vi "Tosca-Clear Digital Outputs.vi"(0 "Config path":path, 11 "error in (no error)":errorcluster) -> (15 "error out":errorcluster)   [LabVIEW 2020]
uses:
  TTL VIs/Device Classes/Base Class/TTLControlledDevice.lvclass
  TTL VIs/Device Classes/Base Class/TTLControlledDevice.lvclass/TTLControlledDevice.ctl
  TTL VIs/Device Classes/Base Class/Read Line.vi
  <vilib>/DAQmx/write.llb/DAQmx Write (Digital 1D Bool 1Chan 1Samp).vi
  epl-vi-lib/Utility VIs/File IO VIs/Configuration File Wrapper VIs/Config-Read Key (string).vi
  <vilib>/DAQmx/create/channels.llb/DAQmx Create Channel (DO-Digital Output).vi
  <vilib>/DAQmx/miscellaneous.llb/DAQmx Fill In Error Info.vi
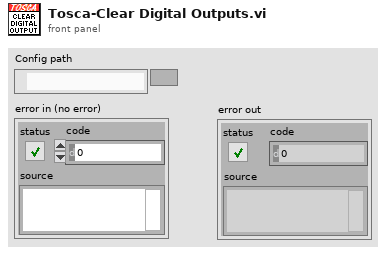
[diagram p1: front panel]
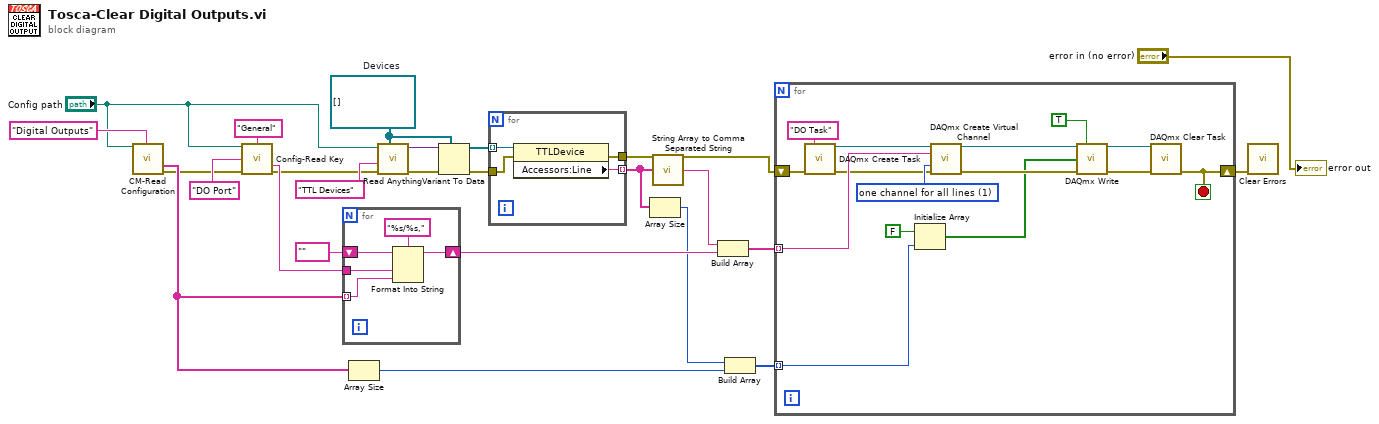
[diagram p0: block diagram]
diagram:
  w15 = refnum<class "TTLControlledDevice.lvclass">[] []  # Devices
  n1 = call "CM-Read Configuration.vi"("Connection File Path"="Config path", "Section"="Digital Outputs") -> ("Devices"=w2:string[], "error out"=w1:errorcluster)  [unwired: 9 in, 3 out]
  n2 = call-poly "Config-Read Key.vi"("configuration file path"="Config path", "section"="General", "key"="DO Port", "error in (no error)"=w1) -> ("value"=w21:string, "error out"=w18:errorcluster)  [unwired: 8 in, 2 out]
  n3 = for {
    tunnel: w2 -> [w26] mode=indexing
    shift-right: [w28] -> w22
    shift-left: tag "" ("DAQmx Physical Channel") -> [w29]
    tunnel: w21 -> [w27]
    n4 = Format Into String(format string="%s/%s,", initial string=w29, w27, w26) -> (resulting string=w28:string)  [unwired: 1 in, 1 out]
  }
  n5 = Array Size(array=w2) -> (size(s)=w20:i32)
  n6 = call "Read Anything.vi"("Type of Anything"=w15, "Error In"=w18, "Section Name (Name of \"Type of Anything\")"="TTL Devices" ("Section Name (Name of \"Type of Anything\")"), "Path (dialog)"="Config path") -> ("Error Out"=w17:errorcluster, "Anything"=w16:variant)  [unwired: 5 in, 1 out]
  n7 = Variant To Data(error in=w17, type=w15, Variant=w16) -> (data=w13:refnum<class "TTLControlledDevice.lvclass">[], error out=w14:errorcluster)
  n8 = for {
    tunnel: w14 -> [w34]
    tunnel: w13 -> [w33] mode=indexing
    tunnel: [w32] -> w10 mode=indexing
    tunnel: [w31] -> w7
    n9 = property class="TTLDevice"(reference=w33, error in=w34) -> (error out=w31:errorcluster, "Accessors:Line"=w32:string)  [unwired: 1 out]
  }
  n10 = Array Size(array=w10) -> (size(s)=w8:i32)
  n11 = call "String Array to Comma Separated String.vi"("String Array"=w10) -> ("comma separated string"=w11:string)
  n12 = Build Array(w11, w22) -> (w12:string[])
  n13 = Build Array(w8, w20) -> (w9:i32[])
  n14 = for {
    tunnel: w12 -> [w49] mode=indexing
    tunnel: w9 -> [w41] mode=indexing
    shift-right: [w35] -> w5
    shift-left: w7 -> [w44]
    stop <- w35 stop-if-true
    w48 = 1 items=["one channel for each line", "one channel for all lines"] ("line grouping")
    n15 = call <vilib>:"DAQmx Create Task.vi"("new task name"="DO Task" ("name to assign"), "error in"=w44) -> ("task out"=w46:refnum<k21>, "error out"=w45:errorcluster)  [unwired: 12 in]
    n16 = Initialize Array(FALSE, w41) -> (w39:bool[])
    n17 = call-poly <vilib>:"DAQmx Create Virtual Channel.vi"("task in"=w46, "lines"=w49, "line grouping"=w48, "error in"=w45) -> ("task out"=w43:refnum<k21>, "error out"=w42:errorcluster)  [unwired: 10 in]
    n18 = call-poly <vilib>:"DAQmx Write.vi"("task/channels in"=w43, "auto start"=TRUE, "data"=w39, "error in"=w42) -> ("task out"=w36:refnum<k21>, "error out"=w37:errorcluster)  [unwired: 9 in, 1 out]
    n19 = call <vilib>:"DAQmx Clear Task.vi"("task in"=w36, "error in"=w37) -> ("error out"=w35:errorcluster)  [unwired: 13 in]
  }
  n20 = call <vilib>:"Clear Errors.vi"("error in (no error)"=w5) -> ()  [unwired: 5 in, 2 out]
  "error out" <- "error in (no error)"
